vi "circle.vi"() -> ()   [LabVIEW 2013]
uses:
  <vilib>/Native 3D Graph/xcontrol/3DPC_SurfacePlot.xctl
  ROS/Code/SubVIs/BaxterSide.ctl
  <vilib>/Analysis/_algsub.llb/Real Vector Norm.vi
  <vilib>/Analysis/baseanly.llb/Real Dot Product.vi
  <vilib>/Analysis/baseanly.llb/A x Vector.vi
  <vilib>/Analysis/Matrix/Numeric/Conversions/Array To Matrix - RA2.vi
  <vilib>/Utility/file.llb/Write To Spreadsheet File (DBL).vi
  <vilib>/Analysis/NI_AALPro.lvlib
  <vilib>/Analysis/NI_AALBase.lvlib
  <vilib>/Analysis/Matrix/NI_Matrix.lvlib
panel:
  in  "Left Arm Offset":dbl=300.0
  out "radius":dbl
  out "3D":refnum<class "Base Datatype.lvclass">[](xcontrol)
  in  "speed":dbl=20.0
  in  "Start":dbl[](array[numeric])=[600.0, -250.0, 0.0]
  in  "Center":dbl[](array[numeric])=[500.0, -250.0, 0.0]
  in  "Axis":dbl[](array[numeric])=[0.0, 0.0, 1.0]
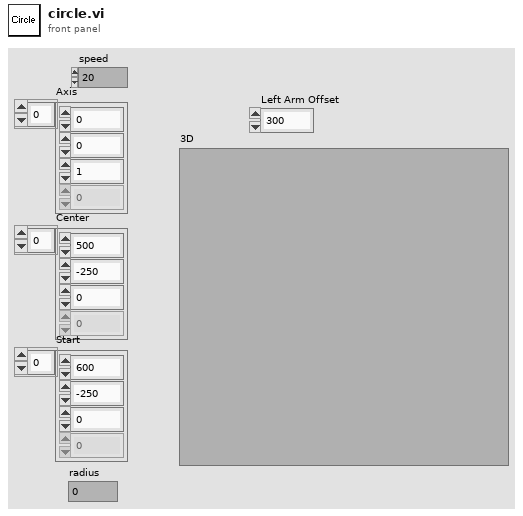
[diagram p1: front panel]
types:
  T1 = typedef "NI_Matrix.lvlib/RealMatrix.ctl" = dbl[][]
  T2 = typedef "BaxterSide.ctl" = enum16{"left", "right"}
  T3 = cluster{"X":dbl, "Y":dbl, "Z":dbl, "Roll":dbl, "Pitch":dbl, "Yaw":dbl}
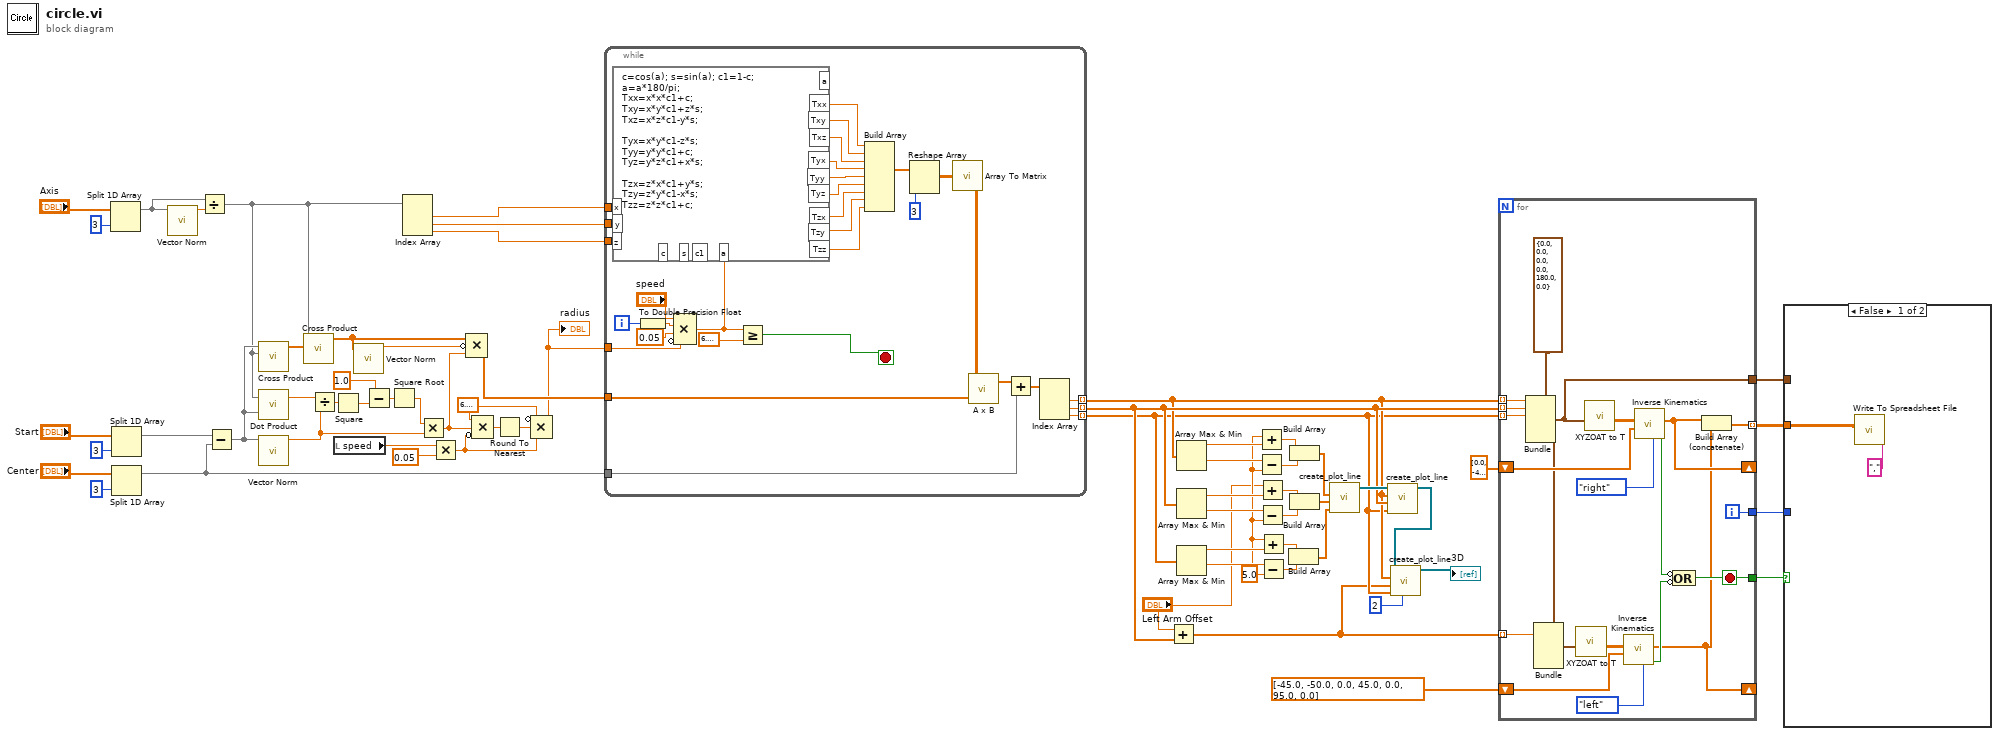
[diagram p0: block diagram]
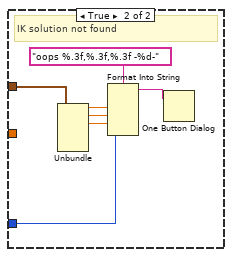
[diagram p2: hidden frame]
diagram:
  w19 = 6.283185307179586
  w33 = 5.0 ("y")
  n1 = Split 1D Array(array="Axis", index=3) -> (first subarray=w58:dbl[])  [unwired: 1 out]
  n2 = Split 1D Array(array="Start", index=3) -> (first subarray=w59:dbl[])  [unwired: 1 out]
  n3 = Split 1D Array(array="Center", index=3) -> (first subarray=w40:dbl[])  [unwired: 1 out]
  n4 = call-poly <vilib>:"Vector Norm.vi"("Input Vector"=w58) -> ("norm"=w57:dbl)  [unwired: 9 in, 1 out]
  n5 = Divide(x=w58, y=w57) -> (x/y=w53:dbl[])
  n6 = Subtract(x=w59, y=w40) -> (x-y=w55:dbl[])
  n7 = call <vilib>:"Cross Product.vi"("B Vector"=w53, "A Vector"=w55) -> ("Cross Product"=w56:dbl[])  [unwired: 8 in, 1 out]
  n8 = call-poly <vilib>:"Dot Product.vi"("Y Vector"=w55, "X Vector"=w53) -> ("X * Y"=w54:dbl)  [unwired: 1 out]
  n9 = call-poly <vilib>:"Vector Norm.vi"("Input Vector"=w55) -> ("norm"=w44:dbl)  [unwired: 9 in, 1 out]
  n10 = call <vilib>:"Cross Product.vi"("B Vector"=w56, "A Vector"=w53) -> ("Cross Product"=w42:dbl[])  [unwired: 8 in, 1 out]
  n11 = Divide(x=w54, y=w44) -> (x/y=w49:dbl)
  n12 = Square(x=w49) -> (x^2=w48:dbl)
  n13 = local read "speed"() -> (w20:dbl)
  n14 = call-poly <vilib>:"Vector Norm.vi"("Input Vector"=w42) -> ("norm"=w41:dbl)  [unwired: 9 in, 1 out]
  n15 = Subtract(x=1.0, y=w48) -> (x-y=w46:dbl)
  n16 = Square Root(x=w46) -> (sqrt(x)=w43:dbl)
  n17 = Index Array(array=w53) -> (element #1=w52:dbl, element #2=w51:dbl, element #3=w50:dbl)  [unwired: 3 in]
  n18 = Multiply(x=w43, y=w44) -> (x*y=w17:dbl)
  n19 = Multiply(x=w20, y=0.05 ("value")) -> (x*y=w18:dbl)
  n20 = Compound Arithmetic op=MULTIPLY(w42, invert w41, w17) -> (w45:dbl[])
  n21 = Compound Arithmetic op=MULTIPLY(w19, w17, invert w18) -> (w22:dbl)
  n22 = Round To Nearest(number=w22) -> (nearest integer value=w15:dbl)
  n23 = Compound Arithmetic op=MULTIPLY(invert w19, w15, w18) -> (w16:dbl)
  "radius" <- w16
  n24 = while {
    tunnel: w52 -> [w96]
    tunnel: w51 -> [w95]
    tunnel: w50 -> [w94]
    tunnel: w16 -> [w81]
    tunnel: w45 -> [w75]
    tunnel: w40 -> [w73]
    tunnel: [w69] -> w3 mode=indexing
    tunnel: [w68] -> w14 mode=indexing
    tunnel: [w67] -> w2 mode=indexing
    i -> [w70]
    stop <- w66 stop-if-true
    w92 = 3 ("dimension size")
    n25 = To Double Precision Float(number=w70) -> (double precision float=w80:dbl)
    n26 = Compound Arithmetic op=MULTIPLY("speed", w80, 0.05 ("value"), invert w81) -> (w77:dbl)
    n27 = formula code="c=cos(a); s=sin(a); c1=1-c;\na=a*180/pi;\nTxx=x*x*c1+c;\nTxy=x*y*c1+z*s;\nTxz=x*z*c1-y*s;\n\nTyx=x*y*c1-z*s;\nTyy=y*y*c1+c;\nTyz=y*z*c1+x*s;\n\nTzx=z*x*c1+y*s;\nTzy=z*y*c1-x*s;\nTzz=z*z*c1+c;"("x"=w96, "y"=w95, "z"=w94, "a"=w77) -> ("Txx"=w90:dbl, "Txy"=w89:dbl, "Txz"=w88:dbl, "Tyx"=w87:dbl, "Tyy"=w86:dbl, "Tyz"=w85:dbl, "Tzx"=w84:dbl, "Tzy"=w83:dbl, "Tzz"=w82:dbl)  [unwired: 4 out]
    n28 = Greater Or Equal?(x=w77, y=6.283185307179586) -> (x >= y?=w66:bool)
    n29 = Build Array(w90, w89, w88, w87, w86, w85, w84, w83, w82) -> (w93:dbl[])
    n30 = Reshape Array(w93, w92, w92) -> (w91:dbl[][])
    n31 = call-poly <vilib>:"Array To Matrix.vi"("Real 2D Array"=w91) -> ("Real Matrix"=w76:T1)
    n32 = call-poly <vilib>:"A x B.vi"("Vector"=w75, "A"=w76) -> ("A x Vector"=w74:dbl[])  [unwired: 1 out]
    n33 = Add(x=w74, y=w73) -> (x+y=w72:dbl[])
    n34 = Index Array(array=w72) -> (element #1=w69:dbl, element #2=w68:dbl, element #3=w67:dbl)  [unwired: 3 in]
  }
  n35 = Add(x="Left Arm Offset", y=w14) -> (x+y=w1:dbl[])
  n36 = Array Max & Min(array=w3) -> (max value=w39:dbl, min value=w38:dbl)  [unwired: 2 out]
  n37 = Array Max & Min(array=w14) -> (max value=w37:dbl, min value=w36:dbl)  [unwired: 2 out]
  n38 = Array Max & Min(array=w2) -> (max value=w34:dbl, min value=w35:dbl)  [unwired: 2 out]
  n39 = Add(x=w33, y=w39) -> (x+y=w32:dbl)
  n40 = Subtract(x=w38, y=w33) -> (x-y=w31:dbl)
  n41 = Add(x="Left Arm Offset", y=w37) -> (x+y=w28:dbl)
  n42 = Subtract(x=w36, y=w33) -> (x-y=w27:dbl)
  n43 = Add(x=w33, y=w34) -> (x+y=w30:dbl)
  n44 = Subtract(x=w35, y=w33) -> (x-y=w29:dbl)
  n45 = Build Array(w30, w29) -> (w24:dbl[])
  n46 = Build Array(w32, w31) -> (w26:dbl[])
  n47 = Build Array(w28, w27) -> (w25:dbl[])
  n48 = call <vilib>:"create_plot_line.vi"("z vector"=w24, "y vector"=w25, "x vector"=w26) -> ("plots out"=w23:refnum<class "Base Datatype.lvclass">[])  [unwired: 2 in, 6 out]
  n49 = call <vilib>:"create_plot_line.vi"("z vector"=w2, "y vector"=w14, "x vector"=w3, "plots in"=w23) -> ("plots out"=w6:refnum<class "Base Datatype.lvclass">[])  [unwired: 1 in, 6 out]
  n50 = call <vilib>:"create_plot_line.vi"("plot ID"=2, "z vector"=w2, "y vector"=w1, "x vector"=w3, "plots in"=w6) -> ("plots out"=→"3D":refnum<class "Base Datatype.lvclass">[])  [unwired: 6 out]
  n51 = for {
    tunnel: w3 -> [w115] mode=indexing
    tunnel: w14 -> [w114] mode=indexing
    tunnel: w2 -> [w113] mode=indexing
    shift-right: [w99] -> _
    shift-left: dbl[] [0.0, -45.0, 0.0, 45.0, 0.0, 90.0, 0.0] ("Start") -> [w112]
    tunnel: [w97] -> w10 mode=indexing
    tunnel: [w103] -> w11
    tunnel: [w110] -> w9
    tunnel: [w108] -> w8
    tunnel: w1 -> [w107] mode=indexing
    shift-right: [w98] -> _
    shift-left: dbl[] [-45.0, -50.0, 0.0, 45.0, 0.0, 95.0, 0.0] ("Joints") -> [w101]
    i -> [w110]
    stop <- w103 stop-if-true
    n52 = Bundle(cluster=T3 {"X"=0.0, "Y"=0.0, "Z"=0.0, "Roll"=0.0, "Pitch"=180.0, "Yaw"=0.0} ("XYZOAT"), "X"=w115, "Y"=w114, "Z"=w113) -> (w108:T3)  [unwired: 3 in]
    n53 = Bundle(cluster=w108, "Y"=w107) -> (w106:T3)  [unwired: 5 in]
    n54 = call "XYZOAT to T.vi"("XYZOAT"=w106) -> ("T"=w105:T1)  [unwired: 10 in]
    n55 = call "XYZOAT to T.vi"("XYZOAT"=w108) -> ("T"=w116:T1)  [unwired: 10 in]
    n56 = call "Inverse Kinematics.vi"("Side"=BaxterSide."left", "Start"=w101, "Goal-matrix"=w105) -> ("Found"=w102:bool, "J"=w98:dbl[])  [unwired: 5 in, 2 out]
    n57 = call "Inverse Kinematics.vi"("Side"=BaxterSide."right", "Start"=w112, "Goal-matrix"=w116) -> ("Found"=w100:bool, "J"=w99:dbl[])  [unwired: 5 in, 2 out]
    n58 = Compound Arithmetic op=OR(invert w100, invert w102) -> (w103:bool)
    n59 = Build Array (concatenate)(w99, w98) -> (w97:dbl[])
  }
  n60 = case shown="False" w11 {
    tunnel: w10 -> [w118 _]
    tunnel: w9 -> [_ w122]
    tunnel: w8 -> [_ w125]
    frame False {
      n61 = call-poly <vilib>:"Write To Spreadsheet File.vi"("delimiter (\\t)"="," ("delimiter (\\t)"), "2D data"=w118) -> ()  [unwired: 6 in, 1 out]
    }
    frame True {
      # "IK solution not found"
      n62 = Unbundle(w125) -> ("X"=w124:dbl, "Y"=w121:dbl, "Z"=w120:dbl)  [unwired: 3 out]
      n63 = Format Into String(format string="oops %.3f,%.3f,%.3f -%d-", w124, w121, w120, w122) -> (resulting string=w119:string)  [unwired: 2 in, 1 out]
      n64 = One Button Dialog(message=w119) -> ()  [unwired: 1 in, 1 out]
    }
  }
